vi "MH_TTraceToGraph.vi"(7 "DeltaT":dbl caption="dt / ms:" format="%.2f", 9 "TimeTrace":u32[][](array[numeric]), 10 "Bin":i32, 11 "Total bin":u64) -> (0 "TimeTrace_out":u32[][](array[numeric]), 1 "dt":dbl, 2 "T0":dbl)   [LabVIEW 2020]
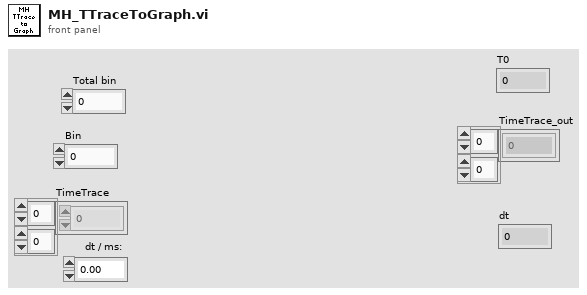
[diagram p1: front panel]
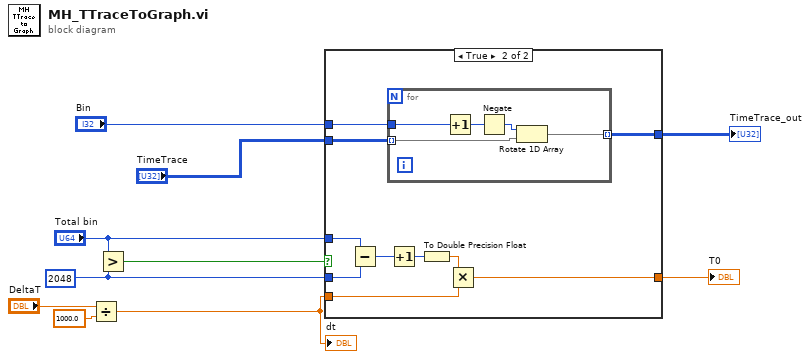
[diagram p0: block diagram]
diagram:
  w1 = u64 2048 ("y")
  n1 = Divide(x="DeltaT", y=1000.0) -> (x/y=w2:dbl)
  "dt" <- w2
  n2 = Greater?(x="Total bin", y=w1) -> (0:w9:bool)
  n3 = case shown="True" w9 {
    tunnel: "Total bin" -> [_ w16]
    tunnel: w2 -> [_ w21]
    tunnel: [_ w20] -> w10
    tunnel: "Bin" -> [_ w18]
    tunnel: "TimeTrace" -> [w11 w12]
    tunnel: [w11 w19] -> w6
    tunnel: w1 -> [_ w13]
    frame False {
    }
    frame True {
      n4 = Subtract(x=w16, y=w13) -> (x-y=w15:u64)
      n5 = for {
        tunnel: [w24] -> w19 mode=indexing
        tunnel: w18 -> [w23]
        tunnel: w12 -> [w22] mode=indexing
        n6 = Increment(x=w23) -> (x+1=w25:i32)
        n7 = Negate(x=w25) -> (-x=w26:i32)
        n8 = Rotate 1D Array(1:w22, 2:w26) -> (0:w24:u32[])
      }
      n9 = Increment(x=w15) -> (x+1=w14:u64)
      n10 = To Double Precision Float(number=w14) -> (double precision float=w17:dbl)
      n11 = Multiply(x=w17, y=w21) -> (x*y=w20:dbl)
    }
  }
  "TimeTrace_out" <- w6
  "T0" <- w10
